vi "Emerson 5700 Units.vi"(8 "Error In":errorcluster, 11 "Emerson Flow Meter Data Input":T1) -> (0 "Error Out":errorcluster, 1 "Basic Units":string[](array[string]), 2 "Units with Mean, STD, ect":string[](array[string]), 3 "Emerson Flow Meter Data Output":T1)   [LabVIEW 2020]
uses:
  Type Definitions/Emerson 5700 Data.ctl
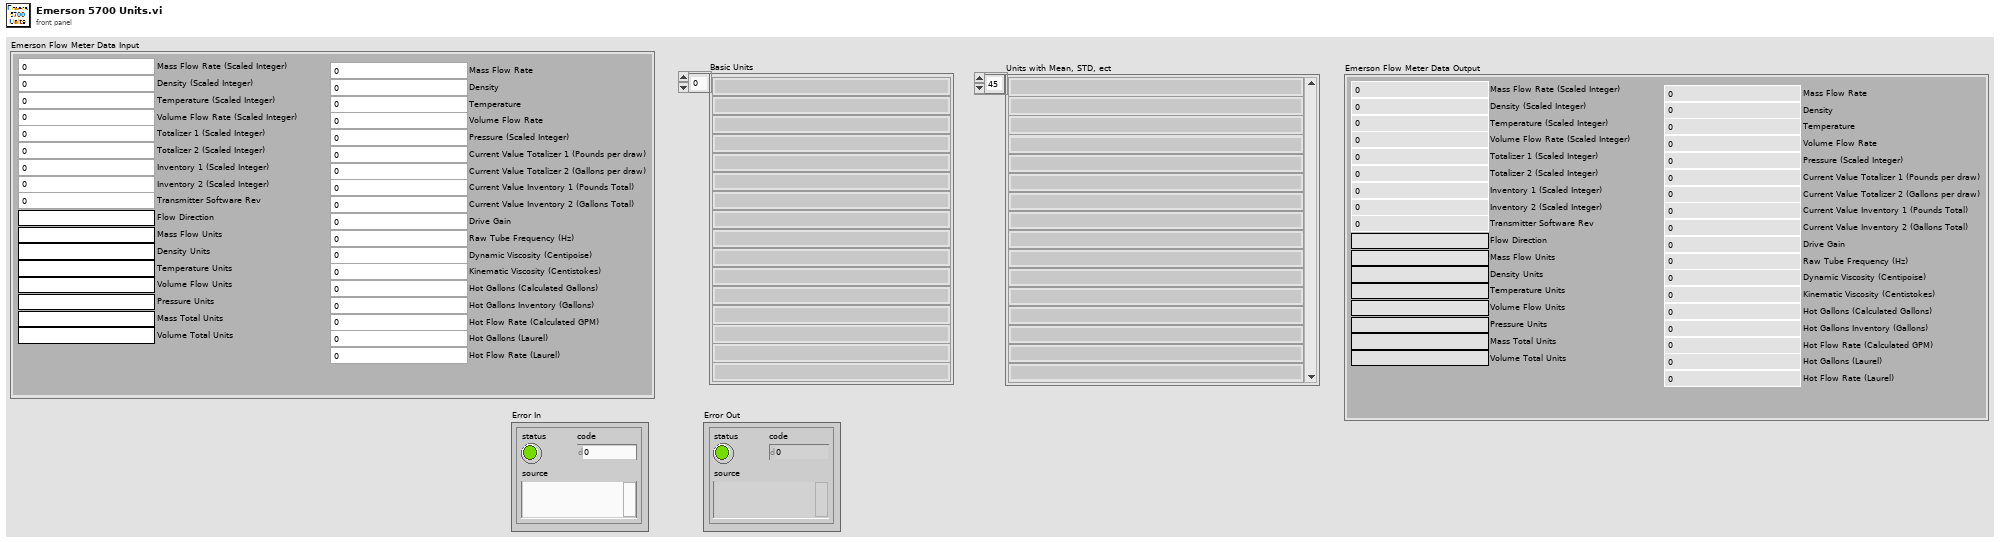
[diagram p1: front panel]
types:
  T1 = typedef "Emerson 5700 Data.ctl" = cluster{"Mass Flow Rate (Scaled Integer)":u16, "Density (Scaled Integer)":u16, "Temperature (Scaled Integer)":u16, "Volume Flow Rate (Scaled Integer)":u16, "Totalizer 1 (Scaled Integer)":u16, "Totalizer 2 (Scaled Integer)":u16, "Transmitter Software Rev":u16, "Flow Direction":string, "Mass Flow Units":string, "Density Units":string, "Temperature Units":string, "Volume Flow Units":string, "Pressure Units":string, "Mass Total Units":string, "Volume Total Units":string, "Inventory 1 (Scaled Integer)":u16, "Inventory 2 (Scaled Integer)":u16, "Mass Flow Rate":dbl, "Density":dbl, "Temperature":dbl, "Volume Flow Rate":dbl, "Pressure (Scaled Integer)":u16, "Current Value Totalizer 1 (Pounds per draw)":dbl, "Current Value Totalizer 2 (Gallons per draw)":dbl, "Current Value Inventory 1 (Pounds Total)":dbl, "Current Value Inventory 2 (Gallons Total)":dbl, "Drive Gain":dbl, "Raw Tube Frequency (Hz)":dbl, "Dynamic Viscosity (Centipoise)":dbl, "Kinematic Viscosity (Centistokes)":dbl, "Hot Gallons (Calculated Gallons)":dbl, "Hot Flow Rate (Calculated GPM)":dbl, "Hot Gallons Inventory (Gallons)":dbl, "Hot Flow Rate (Laurel)":dbl, "Hot Gallons (Laurel)":dbl}
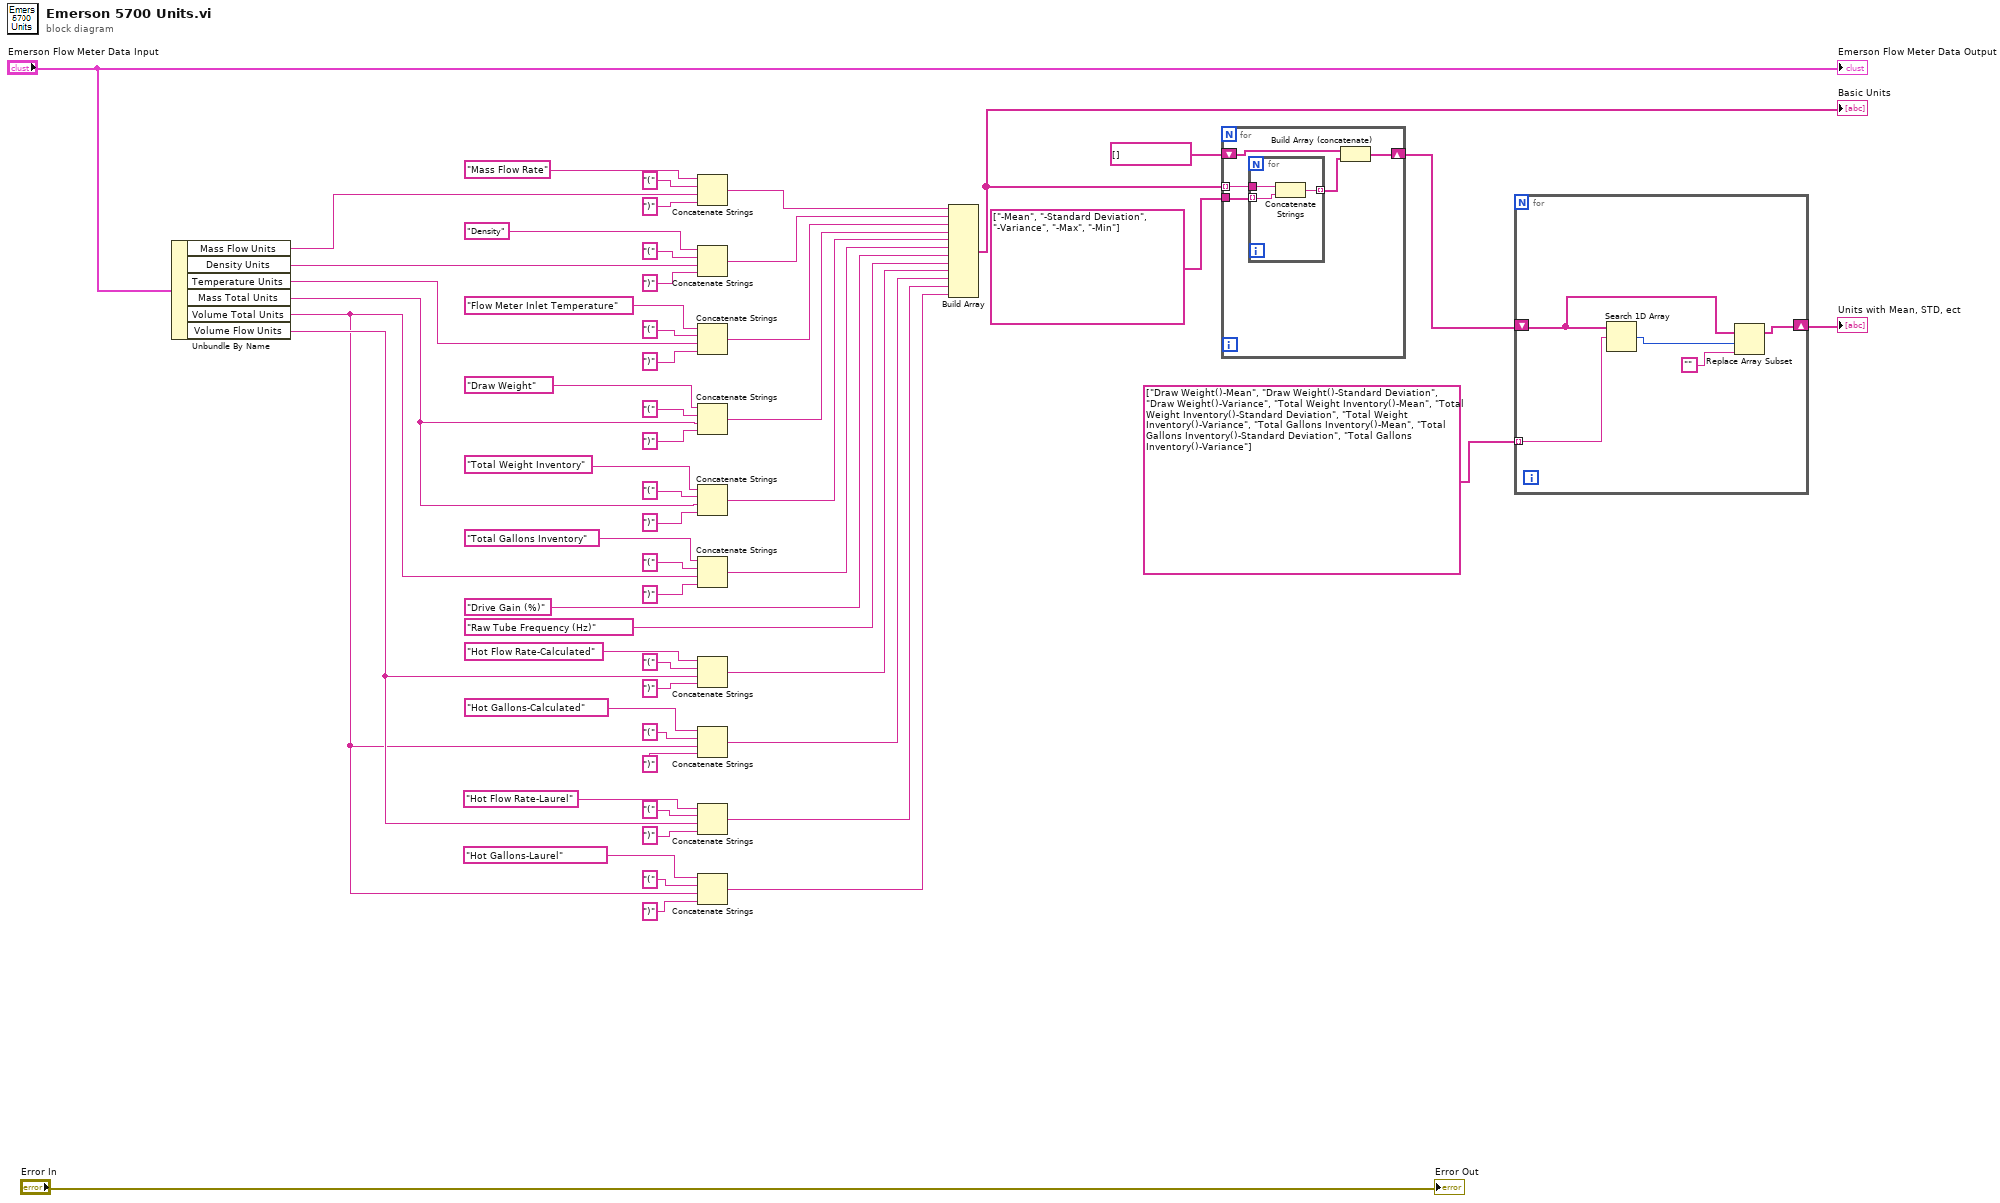
[diagram p0: block diagram]
diagram:
  n1 = Unbundle By Name("Emerson Flow Meter Data Input") -> ("Mass Flow Units"=w53:string, "Density Units"=w54:string, "Temperature Units"=w55:string, "Mass Total Units"=w56:string, "Volume Total Units"=w3:string, "Volume Flow Units"=w4:string)
  n2 = Concatenate Strings("Mass Flow Rate", "(" ("string"), w53, ")" ("string")) -> (w44:string)
  n3 = Concatenate Strings("Density", "(" ("string"), w54, ")" ("string")) -> (w45:string)
  n4 = Concatenate Strings("Flow Meter Inlet Temperature", "(" ("string"), w55, ")" ("string")) -> (w46:string)
  n5 = Concatenate Strings("Draw Weight", "(" ("string"), w56, ")" ("string")) -> (w47:string)
  n6 = Concatenate Strings("Total Weight Inventory", "(" ("string"), w56, ")" ("string")) -> (w48:string)
  n7 = Concatenate Strings("Total Gallons Inventory", "(" ("string"), w3, ")" ("string")) -> (w49:string)
  n8 = Concatenate Strings("Hot Flow Rate-Calculated", "(" ("string"), w4, ")" ("string")) -> (w12:string)
  n9 = Concatenate Strings("Hot Gallons-Calculated", "(" ("string"), w3, ")" ("string")) -> (w11:string)
  n10 = Concatenate Strings("Hot Flow Rate-Laurel", "(" ("string"), w4, ")" ("string")) -> (w2:string)
  n11 = Concatenate Strings("Hot Gallons-Laurel", "(" ("string"), w3, ")" ("string")) -> (w1:string)
  n12 = Build Array(w44, w45, w46, w47, w48, w49, "Drive Gain (%)", "Raw Tube Frequency (Hz)", w12, w11, w2, w1) -> (w25:string[])
  "Basic Units" <- w25
  n13 = for {
    tunnel: w25 -> [w61] mode=indexing
    tunnel: string[] ["-Mean", "-Standard Deviation", "-Variance", "-Max", "-Min"] -> [w60]
    shift-right: [w57] -> w21
    shift-left: string[] [] -> [w59]
    n14 = for {
      tunnel: w61 -> [w64]
      tunnel: w60 -> [w63] mode=indexing
      tunnel: [w62] -> w58 mode=indexing
      n15 = Concatenate Strings(w64, w63) -> (w62:string)
    }
    n16 = Build Array (concatenate)(w59, w58) -> (w57:string[])
  }
  n17 = for {
    tunnel: string[] ["Draw Weight()-Mean", "Draw Weight()-Standard Deviation", "Draw Weight()-Variance", "Total Weight Inventory()-Mean", "Total Weight Inventory()-Standard Deviation", "Total Weight Inventory()-Variance", "Total Gallons Inventory()-Mean", "Total Gallons Inventory()-Standard Deviation", "Total Gallons Inventory()-Variance"] -> [w69] mode=indexing
    shift-right: [w65] -> w19
    shift-left: w21 -> [w68]
    n18 = Search 1D Array(1D array=w68, element=w69) -> (index of element=w67:i32)  [unwired: 1 in]
    n19 = Replace Array Subset(array=w68, new element="", index=w67) -> (w65:string[])
  }
  "Units with Mean, STD, ect" <- w19
  "Error Out" <- "Error In"
  "Emerson Flow Meter Data Output" <- "Emerson Flow Meter Data Input"
